vi "WaitForTime.vi"() -> ()   [LabVIEW 2017]
uses:
  Framework/Robot Global Data.vi
panel:
  in  "Time":dbl
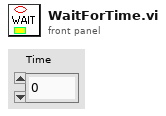
[diagram p1: front panel]
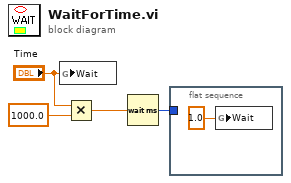
[diagram p0: block diagram]
diagram:
  n1 = global write "Robot Global Data.vi" "Wait"("Time") -> ()
  n2 = Multiply(x="Time", y=1000.0) -> (x*y=w2:dbl)
  n3 = Wait (ms)(milliseconds to wait=w2) -> (millisecond timer value=w1:u32)
  n4 = flat-sequence {
    tunnel: w1 -> [_]
    frame #0 {
      n5 = global write "Robot Global Data.vi" "Wait"(1.0 ("Wait")) -> ()
    }
  }
